vi "SigInfo WfmToMZSpectrum.vi"(8 "error in (no error)":errorcluster, 9 "SectionalSignal":waveform(sgl)) -> (0 "error out":errorcluster, 1 "MassSpectrum":cluster{"X":dbl[], "Y":sgl[]}, 4 "beta":dbl[](array[numeric]))   [LabVIEW 2018, in "SigInfo.lvclass"]
uses:
  SigInfo.lvclass
  SigInfo.lvclass/SigInfo.ctl
  <vilib>/gmath/NI_Gmath.lvlib
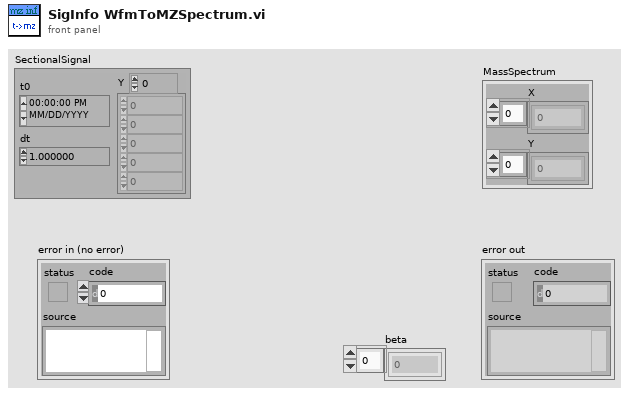
[diagram p1: front panel]
types:
  T1 = cluster{"Label":string, "dt":dbl, "Length":u32, "RefVolt":dbl, "mzTable":cluster{"t":dbl[], "mz":dbl[], "beta":dbl[]}}[]
  T2 = cluster{"Label":string, "dt":dbl, "Length":u32, "RefVolt":dbl, "mzTable":cluster{"t":dbl[], "mz":dbl[], "beta":dbl[]}}
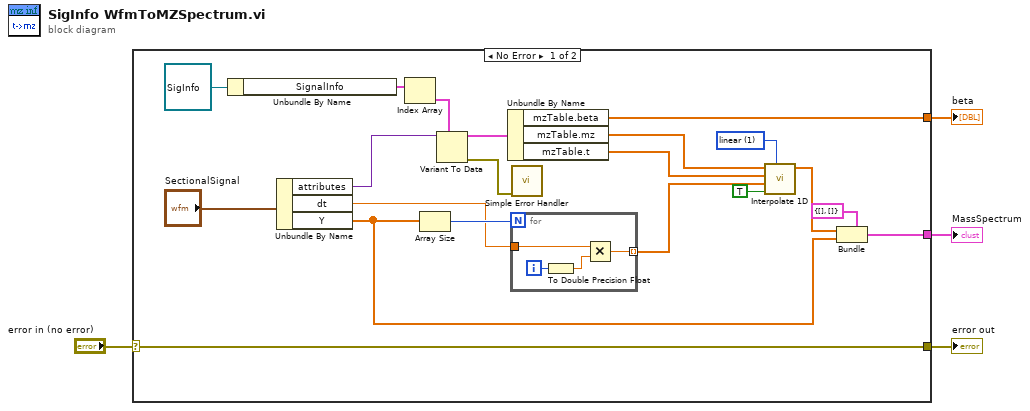
[diagram p0: block diagram]
diagram:
  n1 = case shown="No Error" "error in (no error)" {
    selector: "error in (no error)" -> [w24 w29]
    tunnel: [w24 w29] -> w4
    tunnel: [w17 _] -> w2
    tunnel: [w5 _] -> w1
    frame No Error {
      w23 = 1 items=["nearest", "linear", "spline", "cubic Hermite", "Lagrange"] ("method")
      n2 = Unbundle By Name(refnum<class "SigInfo.lvclass"> refnum ("SigInfo.lvclass")) -> ("SignalInfo"=w15:T1)
      n3 = Unbundle By Name("SectionalSignal") -> ("attributes"=w13:variant, "dt"=w7:dbl, "Y"=w9:sgl[])
      n4 = Index Array(array=w15) -> (element=w14:T2)  [unwired: 1 in]
      n5 = Array Size(array=w9) -> (size(s)=w8:i32)
      n6 = Variant To Data(type=w14, Variant=w13) -> (data=w12:T2, error out=w6:errorcluster)  [unwired: 1 in]
      n7 = Unbundle By Name(w12) -> ("mzTable.beta"=w5:dbl[], "mzTable.mz"=w11:dbl[], "mzTable.t"=w10:dbl[])
      n8 = for {
        N: w8 -> [_]
        tunnel: w7 -> [w26]
        tunnel: [w25] -> w21 mode=indexing
        i -> [w28]
        n9 = To Double Precision Float(number=w28) -> (double precision float=w27:dbl)
        n10 = Multiply(x=w26, y=w27) -> (x*y=w25:dbl)
      }
      n11 = call <vilib>:"Simple Error Handler.vi"("error in (no error)"=w6) -> ()  [unwired: 4 in, 5 out]
      n12 = call <vilib>:"Interpolate 1D.vi"("method"=w23, "X is monotonic"=TRUE, "xi"=w21, "X"=w10, "Y"=w11) -> ("yi"=w20:dbl[])  [unwired: 4 in, 2 out]
      n13 = Bundle(cluster=cluster{"X":dbl[], "Y":sgl[]} {"X"=[], "Y"=[]} ("MassSpectrum 2"), "X"=w20, "Y"=w9) -> (w17:cluster{"X":dbl[], "Y":sgl[]})
    }
    frame Error {
    }
  }
  "error out" <- w4
  "MassSpectrum" <- w2
  "beta" <- w1
